vi "setOnTheFlyPositionChange.vi"(0 "SingleAxisController in":refnum<class "_SingleAxisController.lvclass">, 2 "axis (nc -for multi-axis applications only)":T1, 3 "target_position":i32, 5 "error in (no error)":errorcluster) -> (14 "SingleAxisController out":refnum<class "_SingleAxisController.lvclass">, 17 "success?":bool, 18 "response":string, 19 "error out":errorcluster)   [LabVIEW 2020, in "classes.lvlib" / "_SingleAxisController.lvclass"]
doc: "Produced By:\n\n<B>Kod Integrations, LLC</B>\n4835 Marianne Drive\nMount Airy, MD 21771\nhttp://www.kodintegrations.com\nemail: info@kodintegrations.com\nphone: (240) 687-1288"
uses:
  _SingleAxisController.lvclass
  C:/GEECS/Developers Version/source/Device Drivers/Newmark-NSC-A/Arcus Driver 3.0.0/ArcusUsbComm/classes/Controller/_Controller.lvclass
  axis.ctl
  _Controller.lvclass
  common.lvlib
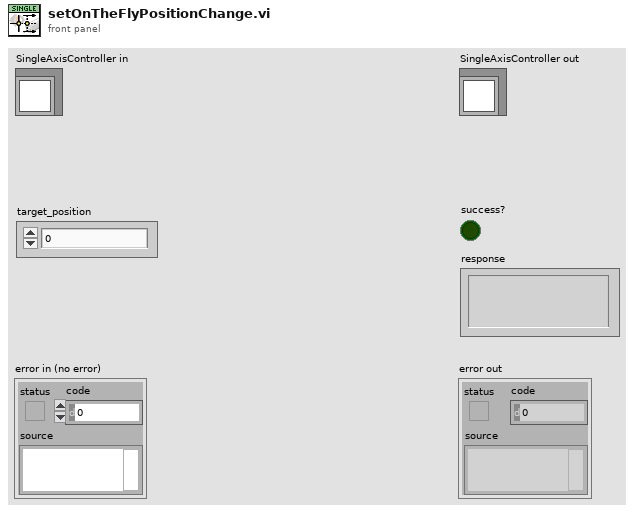
[diagram p1: front panel]
types:
  T1 = typedef "common.lvlib/axis.ctl" = enum16{"X", "Y", "Z", "U"}
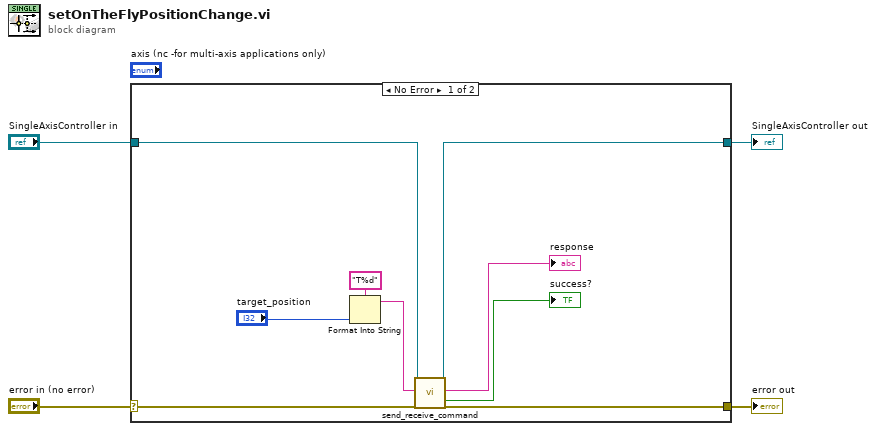
[diagram p0: block diagram]
diagram:
  n1 = case shown="No Error" "error in (no error)" {
    selector: "error in (no error)" -> [w13 w15]
    tunnel: [w12 w15] -> w3
    tunnel: [w8 w14] -> w1
    tunnel: "SingleAxisController in" -> [w9 w14]
    frame No Error {
      n2 = Format Into String(format string="T%d", "target_position") -> (resulting string=w5:string)  [unwired: 2 in, 1 out]
      n3 = call "send_receive_command.vi"("reference (in)"=w9, "ASCII Command (in)"=w5, "error in (no error)"=w13) -> ("reference (out)"=w8:refnum<class "_SingleAxisController.lvclass">, "response (out)"=→"response":string, "success?"=→"success?":bool, "error out"=w12:errorcluster)  [unwired: 12 in, 1 out]
    }
    frame Error {
    }
  }
  "error out" <- w3
  "SingleAxisController out" <- w1
